vi "Tested Information.vi"() -> ()   [LabVIEW 2022 SP3]
uses:
  Axis New Value.ctl
  MAS.lvclass
panel:
  out "Position":dbl[](array[numeric])
  in  "Stop":bool
  out "XY Graph":cluster{"X":dbl, "Y":dbl}[](graph)
  out "error out":errorcluster
  out "Position 2":dbl[](array[numeric])
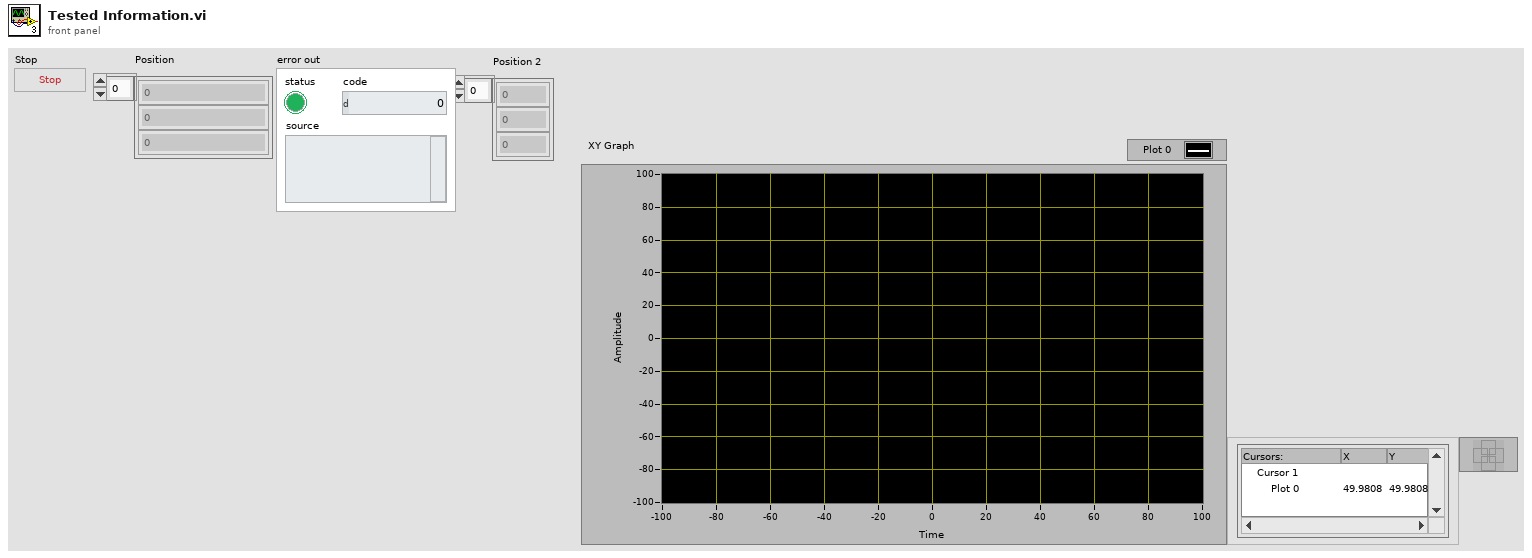
[diagram p1: front panel]
types:
  T1 = typedef "MAS.lvclass/Axis New Value.ctl" = cluster{"Axis Name":string, "New Value":dbl}
  T2 = cluster{"Current Position":dbl, "Current Position":dbl}
  T3 = cluster{"Current Position":dbl, "Current Position":dbl}[]
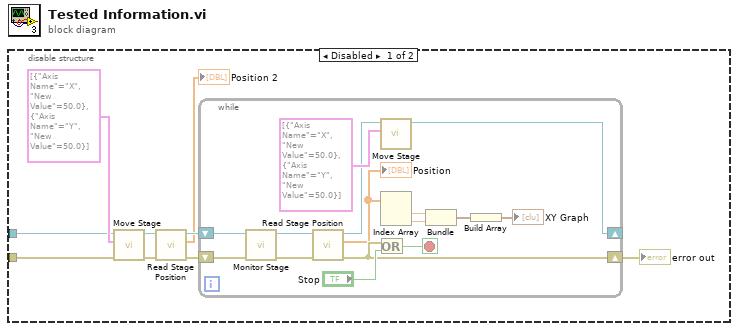
[diagram p0: block diagram]
diagram:
  n1 = disable-structure shown="Disabled" {
    disable-tunnel: _ -> [w8 _]
    disable-tunnel: _ -> [w4 _]
    frame Disabled {
      n2 = call "Move Stage.vi"("error in (no error)"=w4, "Array"=T1[] [{"Axis Name"="X", "New Value"=50.0}, {"Axis Name"="Y", "New Value"=50.0}], "MAS in"=w8) -> ("error out"=w3:errorcluster, "MAS out"=w6:refnum<class "MAS.lvclass">)  [unwired: 7 in]
      n3 = call-dynamic "Read Stage Position.vi"("error in (no error)"=w3, "MAS in"=w6) -> ("error out"=w2:errorcluster, "Position"=→"Position 2":dbl[], "MAS out"=w5:refnum<class "MAS.lvclass">)  [unwired: 7 in]
      n4 = while {
        shift-right: [w10] -> _
        shift-left: w5 -> [w24]
        shift-right: [w18] -> w7
        shift-left: w2 -> [w22]
        stop <- w20 stop-if-true
        n5 = call-dynamic "Monitor Stage.vi"("error in (no error)"=w22, "MAS in"=w24) -> ("error out"=w19:errorcluster, "MAS out"=w23:refnum<class "MAS.lvclass">)  [unwired: 8 in]
        n6 = call-dynamic "Read Stage Position.vi"("error in (no error)"=w19, "MAS in"=w23) -> ("error out"=w18:errorcluster, "Position"=w17:dbl[], "MAS out"=w11:refnum<class "MAS.lvclass">)  [unwired: 7 in]
        "Position" <- w17
        n7 = Or(x=w18, y="Stop") -> (x .or. y?=w20:bool)
        n8 = call "Move Stage.vi"("Array"=T1[] [{"Axis Name"="X", "New Value"=50.0}, {"Axis Name"="Y", "New Value"=50.0}], "MAS in"=w11) -> ("MAS out"=w10:refnum<class "MAS.lvclass">)  [unwired: 8 in, 1 out]
        n9 = Index Array(array=w17) -> (element #1=w16:dbl, element #2=w15:dbl)  [unwired: 2 in]
        n10 = Bundle("Current Position"=w16, "Current Position"=w15) -> (w14:T2)  [unwired: 1 in]
        n11 = Build Array(w14) -> (→"XY Graph":T3)
      }
      "error out" <- w7
    }
    frame Enabled {
    }
  }
